vi "s.vi"() -> ()   [LabVIEW 2017]
uses:
  <vilib>/nican/nican.llb/CanFrameTimed.ctl
panel:
  out "CAN DATA 2":T1[](array[typedef]) {"Data" format="%.0x"; "ArbitrationId" format="%.0x"; "Timestamp" format="%<%I:%M:%S%3u %p\n%m/%d/%Y>T"}
  in  "CAN DATA":T1[](array[typedef]) {"Data" format="%.0x"; "ArbitrationId" format="%.0x"; "Timestamp" format="%<%I:%M:%S%3u %p\n%m/%d/%Y>T"}
  in  "Actual CAN Array":string[][](array[string])
  out "Output Array 2":string[][](array[string])=[["10:43:53.209", "20000688", "CAN Data Frame\r\n", " 8", "64\t41\t00\t00\t00\t00\t00\tA3\r\n", ""], ["10:43:53.189", "20000687", "CAN Data Frame\r\n", " 8", "3D\t00\t00\t00\t00\t00\t00\t51\r\n", ""], ["10:43:53.009", "20000688", "CAN Data Frame\r\n", " 8", "64\t41\t00\t00\t00\t00\t00\t9B\r\n", ""], ["10:43:52.989", "20000687", "CAN Data Frame\r\n", " 8", "3D\t00\t00\t00\t00\t00\t00\t4D\r\n", ""], ["10:43:52.809", "20000688", "CAN Data Frame\r\n", " 8", "64\t41\t00\t00\t00\t00\t00\t93\r\n", ""], ["10:43:52.789", "20000687", "CAN Data Frame\r\n", " 8", "3D\t00\t00\t00\t00\t00\t00\t49\r\n", ""], ["10:43:52.609", "20000688", "CAN Data Frame\r\n", " 8", "64\t41\t00\t00\t00\t00\t00\t8B\r\n", ""], ["10:43:52.589", "20000687", "CAN Data Frame\r\n", " 8", "3D\t00\t00\t00\t00\t00\t00\t45\r\n", ""], ["10:43:52.408", "20000688", "CAN Data Frame\r\n", " 8", "64\t41\t00\t00\t00\t00\t00\t83\r\n", ""], ["10:43:52.388", "20000687", "CAN Data Frame\r\n", " 8", "3D\t00\t00\t00\t00\t00\t00\t41\r\n", ""], ["10:43:52.208", "20000688", "CAN Data Frame\r\n", " 8", "64\t41\t00\t00\t00\t00\t00\t7B\r\n", ""], ["10:43:52.188", "20000687", "CAN Data Frame\r\n", " 8", "3D\t00\t00\t00\t00\t00\t00\t3D\r\n", ""], ["10:43:52.008", "20000688", "CAN Data Frame\r\n", " 8", "64\t41\t00\t00\t00\t00\t00\t73\r\n", ""], ["10:43:51.988", "20000687", "CAN Data Frame\r\n", " 8", "3D\t00\t00\t00\t00\t00\t00\t39\r\n", ""], ["10:43:51.808", "20000688", "CAN Data Frame\r\n", " 8", "64\t41\t00\t00\t00\t00\t00\t6B\r\n", ""]]
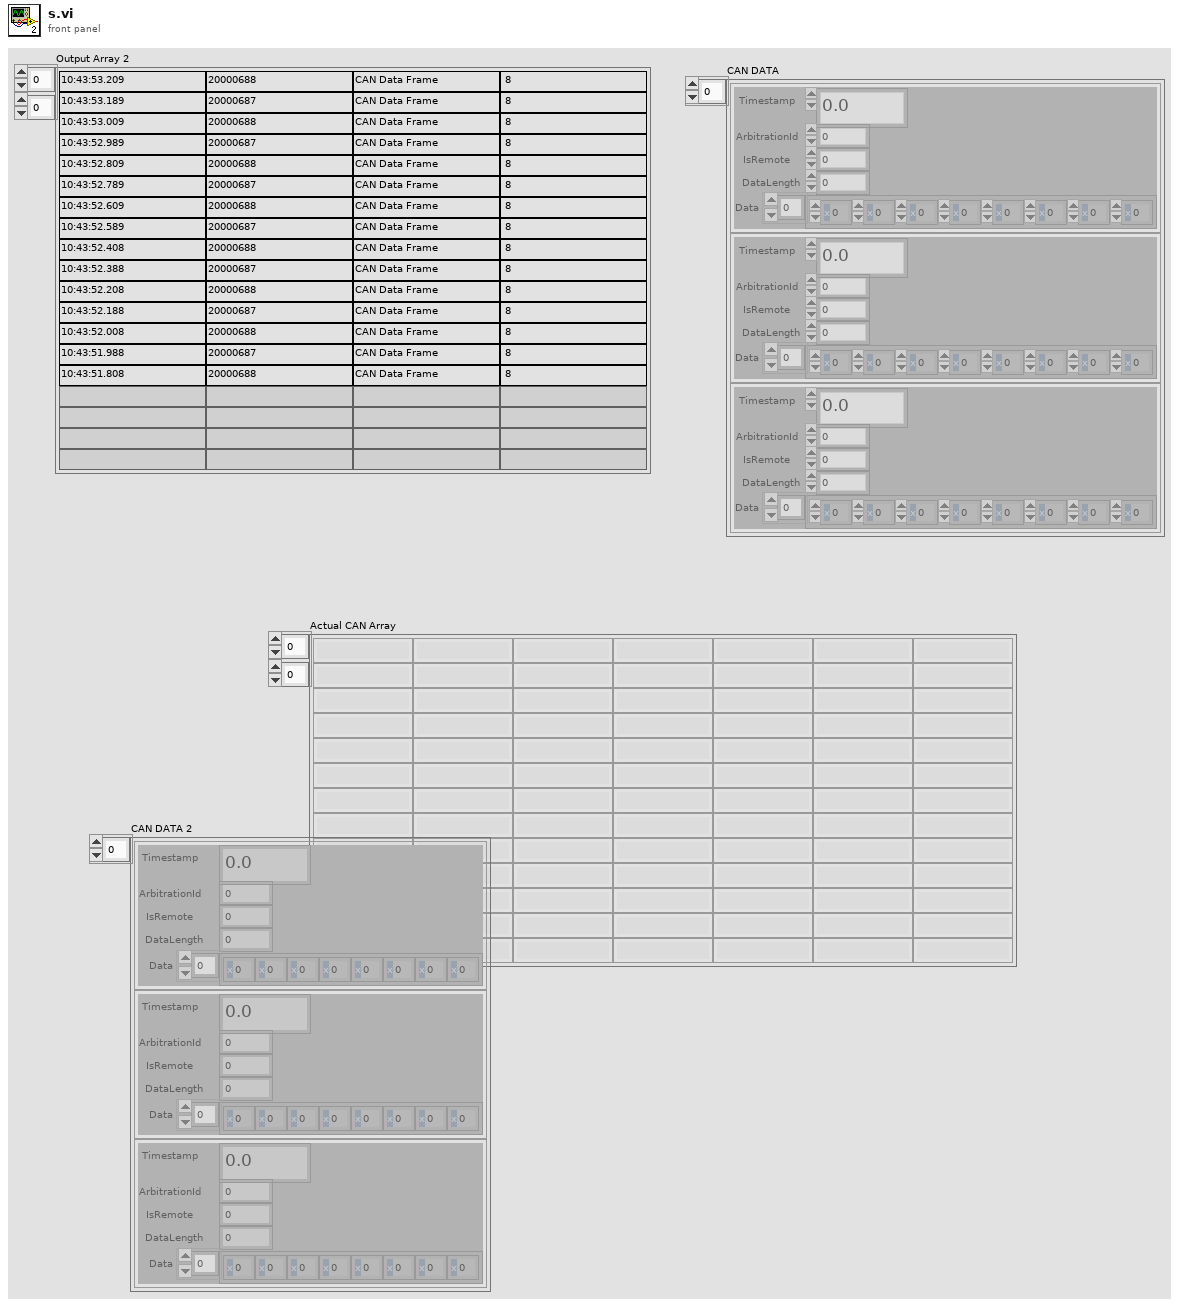
[diagram p1: front panel]
types:
  T1 = typedef "CanFrameTimed.ctl" = cluster{"Timestamp":dbl, "ArbitrationId":u32, "IsRemote":u8, "DataLength":u8, "Data":u8[]}
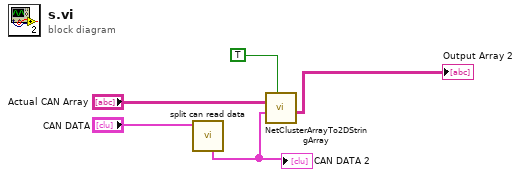
[diagram p0: block diagram]
diagram:
  n1 = call "split can read data.vi"("CAN DATA"="CAN DATA") -> ("CAN DATA 2"=w1:T1[])  [unwired: 6 in, 4 out]
  "CAN DATA 2" <- w1
  n2 = call <vilib>:"NetClusterArrayTo2DStringArray.vi"("Hexadecimal?"=TRUE, "Data from ncReadNetMult"=w1, "Input Array"="Actual CAN Array") -> ("Output Array"=→"Output Array 2":string[][])  [unwired: 8 in]
